vi "auto_script_parser.vi"(7 "Tool Assignments":T1, 10 "Script name in":string="Script_1.txt", 11 "Script folder path":path=path "R:/Programing/Scriping/home/lvuser/auto") -> ()   [LabVIEW 2017, in "labview-standard-library.lvlib" / "automode-scripting.lvlib"]
uses:
  automode-scripting.lvlib
  Footer_cluster.ctl
  type-defs/tool-assignments.ctl
panel:
  in  "Drive subsystem name":string="Drive"
  out "notifications":string[](array[string])
  out "error out":errorcluster
  in  "Footer VI Cluster":T2
  out "File text out":string
  out "text":string
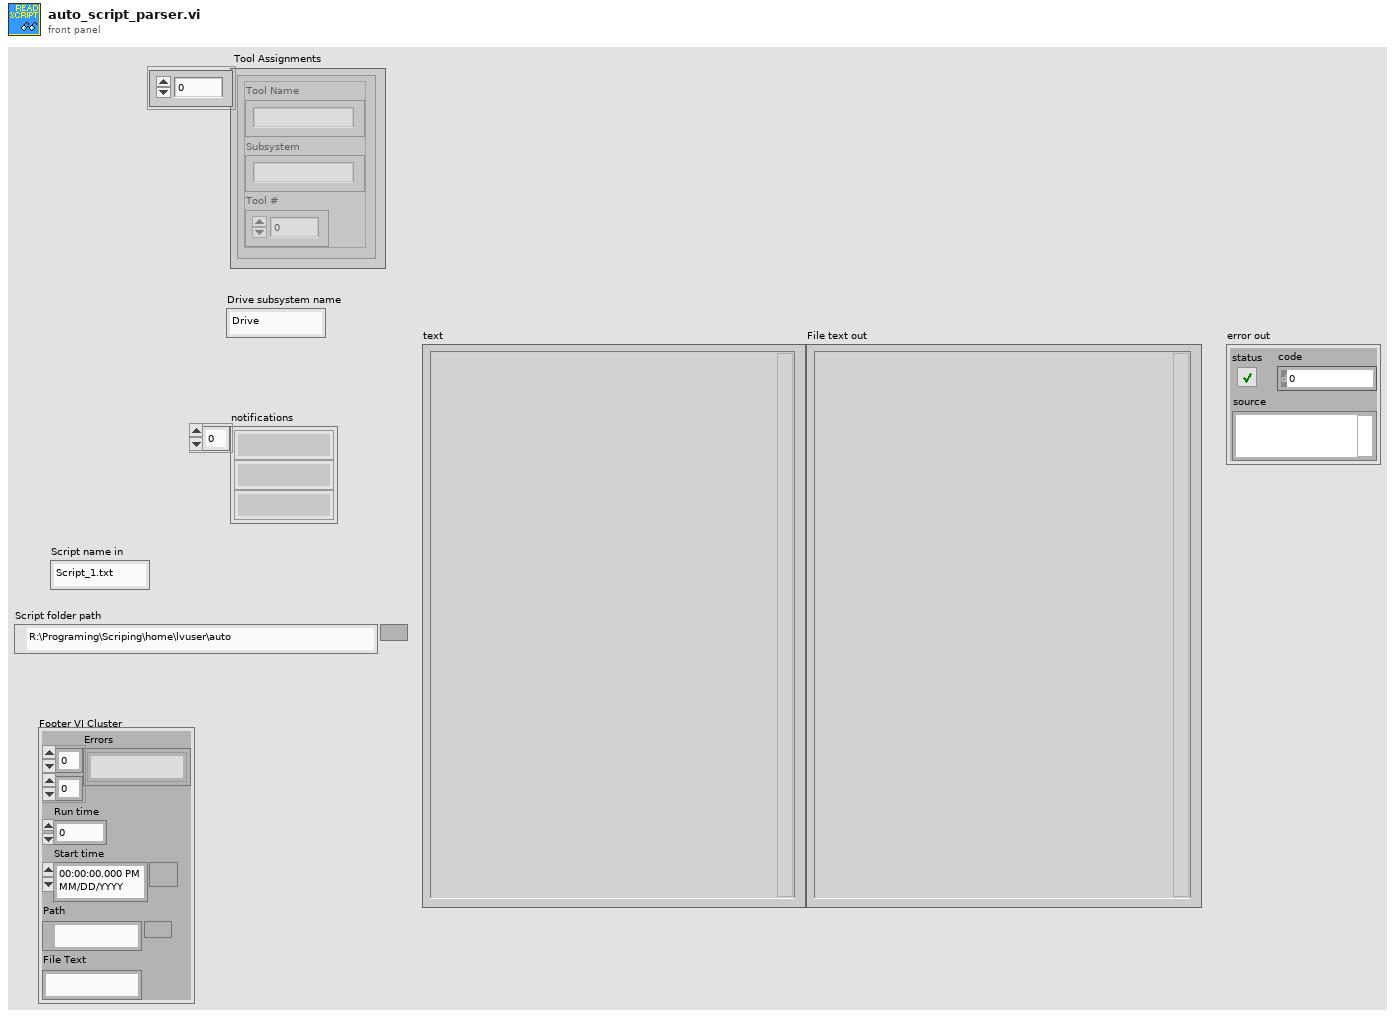
[diagram p1: front panel]
types:
  T1 = typedef "tool-assignments.ctl" = cluster{"Tool Name":string, "Subsystem":string, "Tool #":i32}[]
  T2 = typedef "labview-standard-library.lvlib/automode-scripting.lvlib/Footer_cluster.ctl" = cluster{"Errors":string[][], "Run time":dbl, "Start time":timestamp, "Path":path, "File Text":string}
  T3 = typedef "labview-standard-library.lvlib/automode-scripting.lvlib/code_types.ctl" = enum16{"g1", "g2", "g3", "g4", "g7", "m0", "m2", "tool", "comment"}
  T4 = typedef "labview-standard-library.lvlib/automode-scripting.lvlib/execution_stop_type.ctl" = enum16{"G4 timed pause", "G4 previous line pause", "G4 tool pause", "Invalid"}
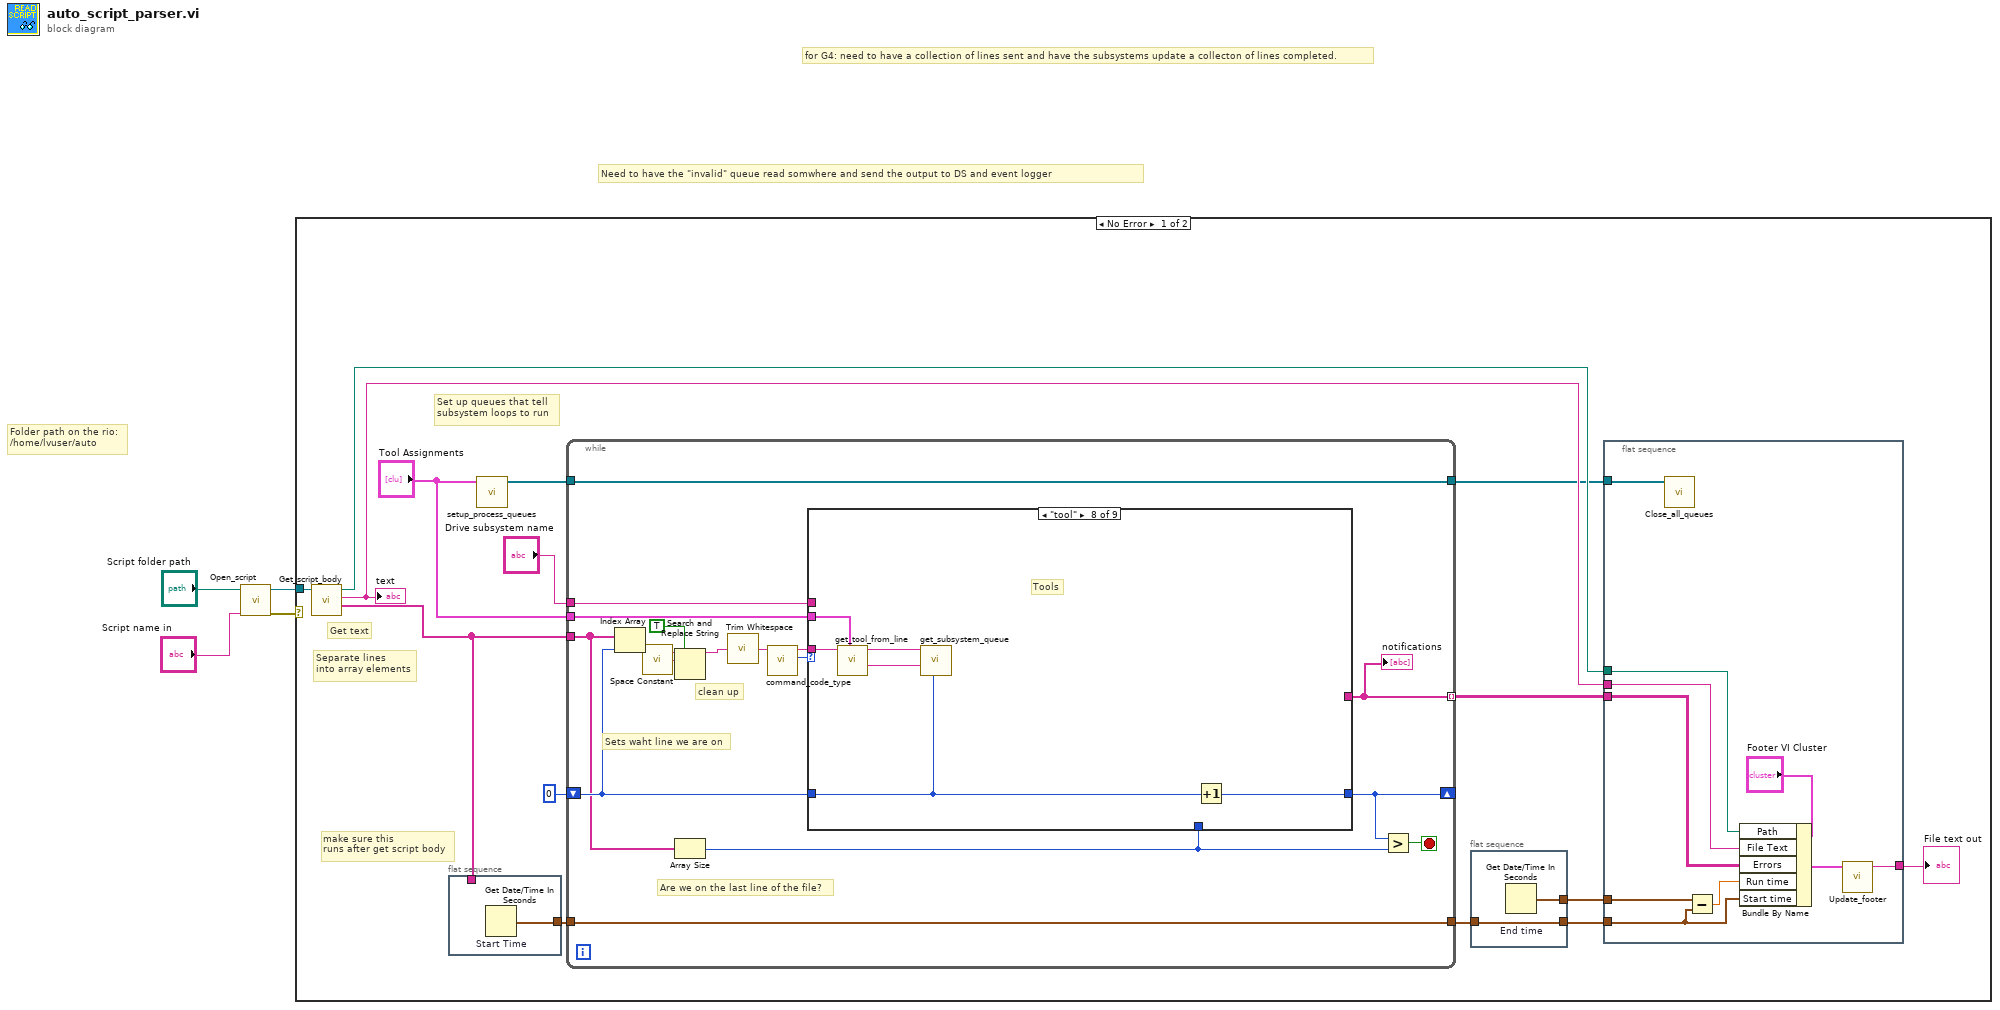
[diagram p0: block diagram]
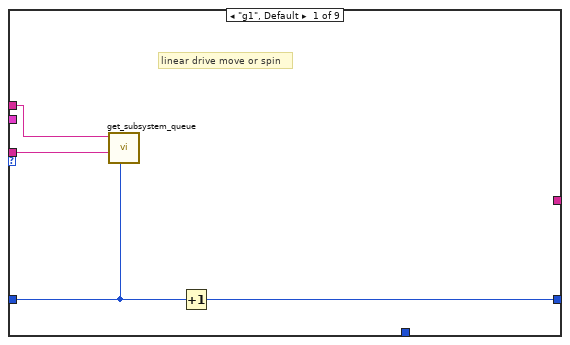
[diagram p2: hidden frame]
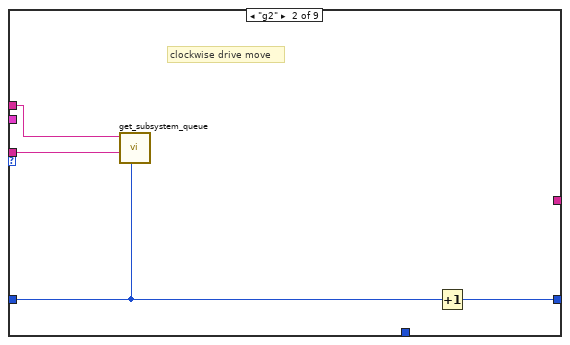
[diagram p3: hidden frame]
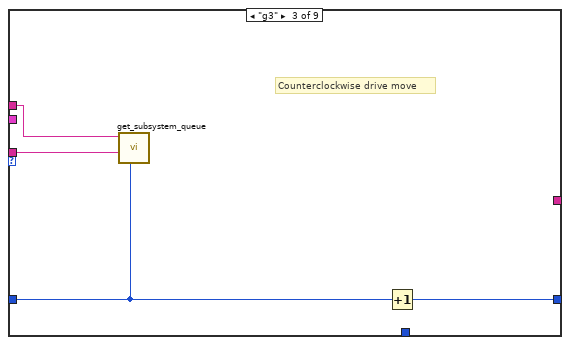
[diagram p4: hidden frame]
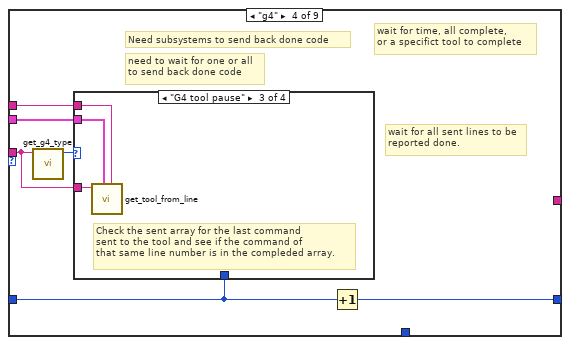
[diagram p5: hidden frame]
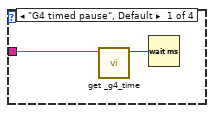
[diagram p6: hidden frame]
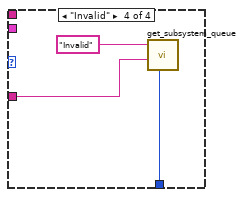
[diagram p8: hidden frame]
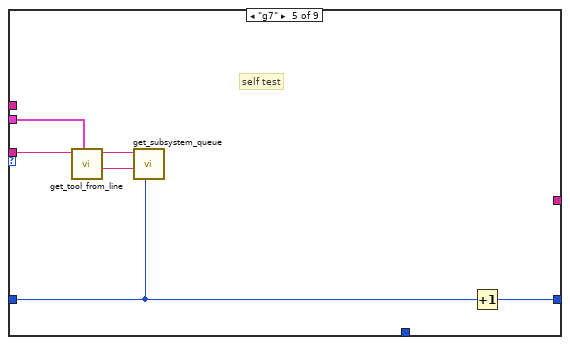
[diagram p9: hidden frame]
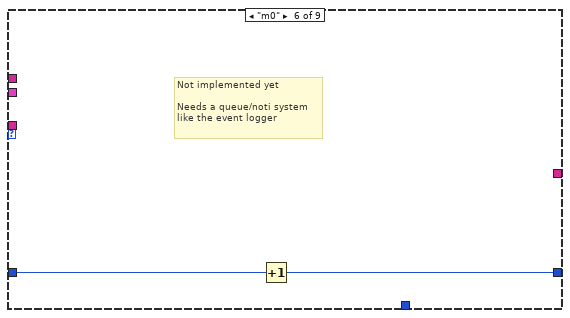
[diagram p10: hidden frame]
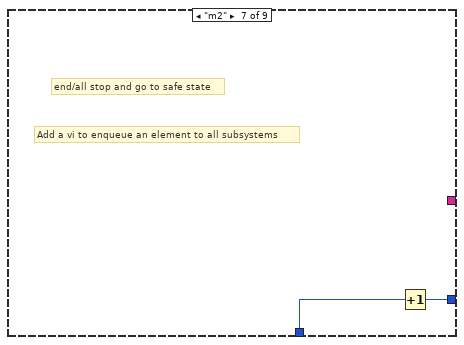
[diagram p11: hidden frame]
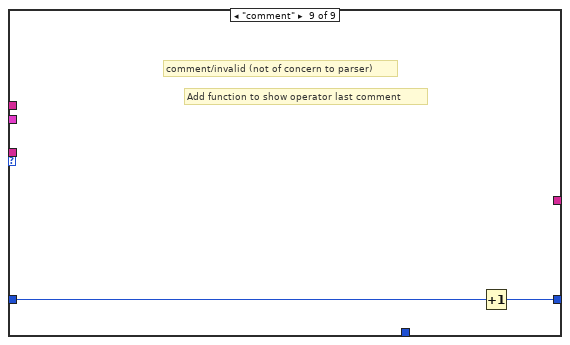
[diagram p12: hidden frame]
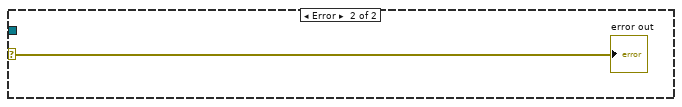
[diagram p13: hidden frame]
diagram:
  # "for G4: need to have a collection of lines sent and have the subsystems update a collecton of lines completed."
  # "Need to have the \"invalid\" queue read somwhere and send the output to DS and event logger"
  # "Folder path on the rio:\n/home/lvuser/auto"
  n1 = call "Open_script.vi"("Script name"="Script name in", "Folder Path"="Script folder path") -> ("error out"=w2:errorcluster, "Byte Stream File out"=w1:refnum<file>)  [unwired: 8 in]
  n2 = case shown="No Error" w2 {
    selector: w2 -> [_ w95]
    tunnel: w1 -> [w18 _]
    frame No Error {
      # "make sure this\nruns after get script body"
      # "Get text"
      # "Set up queues that tell\nsubsystem loops to run"
      # "Separate lines\ninto array elements"
      n3 = call "Get_script_body.vi"("Byte Stream File in"=w18) -> ("Script Body"=w7:string[], "Full Text"=w14:string, "File Path Out"=w16:path)  [unwired: 8 in]
      "text" <- w14
      n4 = flat-sequence {
        tunnel: [w20] -> w17
        tunnel: w7 -> [_]
        frame #0 {
          n5 = Get Date/Time In Seconds "Start Time"() -> (seconds since 1Jan1904=w20:timestamp)
        }
      }
      n6 = call "setup_process_queues.vi"("Tool Assignments"="Tool Assignments") -> ("Process queues"=w12:refnum<queue>[])  [unwired: 9 in, 1 out]
      n7 = while {
        shift-right: [w48] -> _
        shift-left: 0 ("index") -> [w49]
        tunnel: w7 -> [w46]
        tunnel: w17 -> [w45]
        tunnel: [w45] -> w10
        tunnel: [w43] -> w15 mode=indexing
        tunnel: [w44] -> w11
        tunnel: w12 -> [w44]
        tunnel: "Tool Assignments" -> [w34]
        tunnel: "Drive subsystem name" -> [w33]
        stop <- w47 stop-if-true
        # "clean up"
        # "Are we on the last line of the file?"
        # "Sets waht line we are on"
        n8 = Index Array(array=w46, index=w49) -> (element=w38:string)
        n9 = call <vilib>:"Space Constant.vi"() -> ("String"=w40:string)
        n10 = Search and Replace String(replace all?=TRUE ("replace all? (F)"), input string=w38, search string=w40) -> (result string=w37:string)  [unwired: 5 in, 3 out]
        n11 = Array Size(array=w46) -> (size(s)=w35:i32)
        n12 = call <vilib>:"Trim Whitespace.vi"("string"=w37) -> ("trimmed string"=w36:string)  [unwired: 1 in]
        n13 = call "command_code_type.vi"("Line in"=w36) -> ("Code type out"=w42:T3, "Line out"=w41:string)  [unwired: 9 in]
        n14 = case shown="\"tool\"" w42 {
          tunnel: w49 -> [w51 w55 w60 w64 w82 w84 _ w92 w94]
          tunnel: [w53 w57 w59 w68 w81 w83 w85 w91 w93] -> w48
          tunnel: [_ _ _ w67 _ _ _ _ _] -> w43
          tunnel: w41 -> [w52 w56 w61 w65 w80 _ _ w90 _]
          tunnel: w35 -> [_ _ _ _ _ _ w86 _ _]
          tunnel: w34 -> [_ _ _ w63 w79 _ _ w89 _]
          tunnel: w33 -> [w50 w54 w58 w62 _ _ _ _ _]
          frame "g1", Default {
            # "linear drive move or spin"
            n15 = call "get_subsystem_queue.vi"("Line #"=w51, "Line in"=w52, "Subsystem in"=w50) -> ()  [unwired: 9 in]
            n16 = Increment(x=w51) -> (x+1=w53:i32)
          }
          frame "g2" {
            # "clockwise drive move"
            n17 = call "get_subsystem_queue.vi"("Line #"=w55, "Line in"=w56, "Subsystem in"=w54) -> ()  [unwired: 9 in]
            n18 = Increment(x=w55) -> (x+1=w57:i32)
          }
          frame "g3" {
            # "Counterclockwise drive move"
            n19 = call "get_subsystem_queue.vi"("Line #"=w60, "Line in"=w61, "Subsystem in"=w58) -> ()  [unwired: 9 in]
            n20 = Increment(x=w60) -> (x+1=w59:i32)
          }
          frame "g4" {
            # "wait for all sent lines to be\nreported done."
            # "wait for time, all complete,\nor a specifict tool to complete"
            # "need to wait for one or all\nto send back done code"
            # "Need subsystems to send back done code"
            n21 = call "get_g4_type.vi"("Line in"=w65) -> ("G4 type"=w66:T4)  [unwired: 9 in, 1 out]
            n22 = case shown="\"G4 tool pause\"" w66 {
              tunnel: w65 -> [w69 _ w73 w76]
              tunnel: w64 -> [_ _ _ w75]
              tunnel: w63 -> [_ _ w72 _]
              tunnel: w62 -> [_ _ w71 _]
              frame "G4 timed pause", Default {
                n23 = call "get _g4_time.vi"("Line in"=w69) -> ("Time to wait"=w70:u32)  [unwired: 10 in]
                n24 = Wait (ms)(milliseconds to wait=w70) -> ()  [unwired: 1 out]
              }
              frame "G4 previous line pause" {
                # "wait for the last item in the sent array\nto appear in the completed array"
              }
              frame "G4 tool pause" {
                # "Check the sent array for the last command\nsent to the tool and see if the command of\nthat same line number is in the compleded array."
                n25 = call "get_tool_from_line.vi"("Drive subsystem name"=w71, "Tool Assignments"=w72, "line in"=w73) -> ()  [unwired: 7 in, 2 out]
              }
              frame "Invalid" {
                n26 = call "get_subsystem_queue.vi"("Line #"=w75, "Line in"=w76, "Subsystem in"="Invalid") -> ()  [unwired: 9 in]
              }
            }
            n27 = Increment(x=w64) -> (x+1=w68:i32)
          }
          frame "g7" {
            # "self test"
            n28 = call "get_tool_from_line.vi"("Tool Assignments"=w79, "line in"=w80) -> ("line out"=w77:string, "Subsystem out"=w78:string)  [unwired: 8 in]
            n29 = call "get_subsystem_queue.vi"("Line #"=w82, "Line in"=w77, "Subsystem in"=w78) -> ()  [unwired: 9 in]
            n30 = Increment(x=w82) -> (x+1=w81:i32)
          }
          frame "m0" {
            # "Not implemented yet\n\nNeeds a queue/noti system\nlike the event logger"
            n31 = Increment(x=w84) -> (x+1=w83:i32)
          }
          frame "m2" {
            # "Add a vi to enqueue an element to all subsystems"
            # "end/all stop and go to safe state"
            n32 = Increment(x=w86) -> (x+1=w85:i32)
          }
          frame "tool" {
            # "Tools"
            n33 = call "get_tool_from_line.vi"("Tool Assignments"=w89, "line in"=w90) -> ("line out"=w87:string, "Subsystem out"=w88:string)  [unwired: 8 in]
            n34 = call "get_subsystem_queue.vi"("Line #"=w92, "Line in"=w87, "Subsystem in"=w88) -> ()  [unwired: 9 in]
            n35 = Increment(x=w92) -> (x+1=w91:i32)
          }
          frame "comment" {
            # "Add function to show operator last comment"
            # "comment/invalid (not of concern to parser)"
            n36 = Increment(x=w94) -> (x+1=w93:i32)
          }
        }
        "notifications" <- w43
        n37 = Greater?(x=w48, y=w35) -> (0:w47:bool)
      }
      n38 = flat-sequence {
        tunnel: [w22] -> w9
        tunnel: w10 -> [w22]
        tunnel: [w21] -> w8
        frame #0 {
          n39 = Get Date/Time In Seconds "End time"() -> (seconds since 1Jan1904=w21:timestamp)
        }
      }
      n40 = flat-sequence {
        tunnel: w9 -> [w32]
        tunnel: w16 -> [w31]
        tunnel: w15 -> [w30]
        tunnel: w14 -> [w29]
        tunnel: [w28] -> w13
        tunnel: w11 -> [w23]
        tunnel: w8 -> [w24]
        frame #0 {
          n41 = call "Close_all_queues.vi"("Process queues"=w23) -> ()  [unwired: 11 in]
          n42 = Subtract(x=w24, y=w32) -> (x-y=w27:dbl)
          n43 = Bundle By Name(cluster="Footer VI Cluster", "Path"=w31, "File Text"=w29, "Errors"=w30, "Run time"=w27, "Start time"=w32) -> (w25:T2)
          n44 = call "Update_footer.vi"("Footer info"=w25) -> ("File text out"=w28:string)  [unwired: 10 in]
        }
      }
      "File text out" <- w13
    }
    frame Error {
      "error out" <- w95
    }
  }
